vi "HH_Start.vi"(0 "Device Index":i32, 5 "Acq. Time":i32, 11 "error in (no error)":errorcluster) -> (4 "Is Error":bool, 15 "error out":errorcluster)   [LabVIEW 2010]
uses:
  hhlib.dll
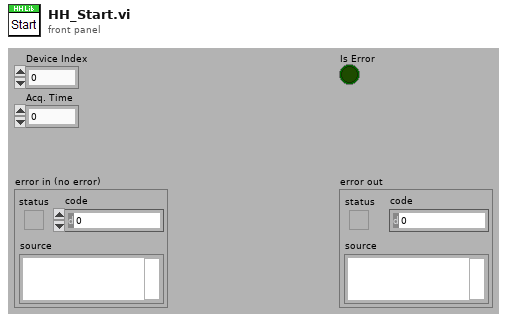
[diagram p1: front panel]
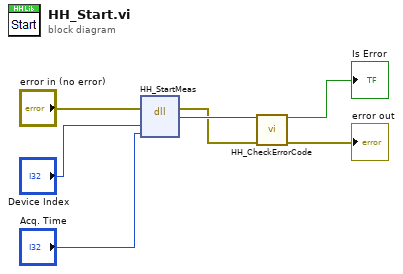
[diagram p0: block diagram]
diagram:
  n1 = dll-call lib="C:/LabVIEW Programs/MT Scan/SubVIs/hhlib.dll" fn="HH_StartMeas"(error in="error in (no error)", "devidx"="Device Index", "tacq"="Acq. Time") -> (error out=w3:errorcluster, "return type"=w4:i32)  [unwired: 4 in, 1 out]
  n2 = call "HH_CheckErrorCode.vi"("errcode"=w4, "error in (no error)"=w3) -> ("Is Error"=→"Is Error":bool, "error out"=→"error out":errorcluster)  [unwired: 12 in]
